vi "Step Index Assigner.vi"(0 "Parameters In":string[][](array[string]), 5 "Controller?":bool=TRUE, 7 "Flow":i32, 9 "Maxes":dbl[](array[numeric]), 11 "Mins":dbl[](array[numeric])) -> (4 "Parameters Out":string[][](array[string]), 6 "Valid?":bool, 8 "TimeValid?":bool, 10 "ProfileValid?":bool, 15 "NoCoerces":bool)   [LabVIEW 2013]
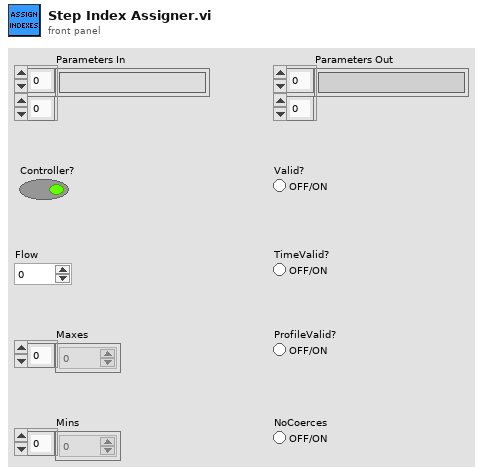
[diagram p1: front panel]
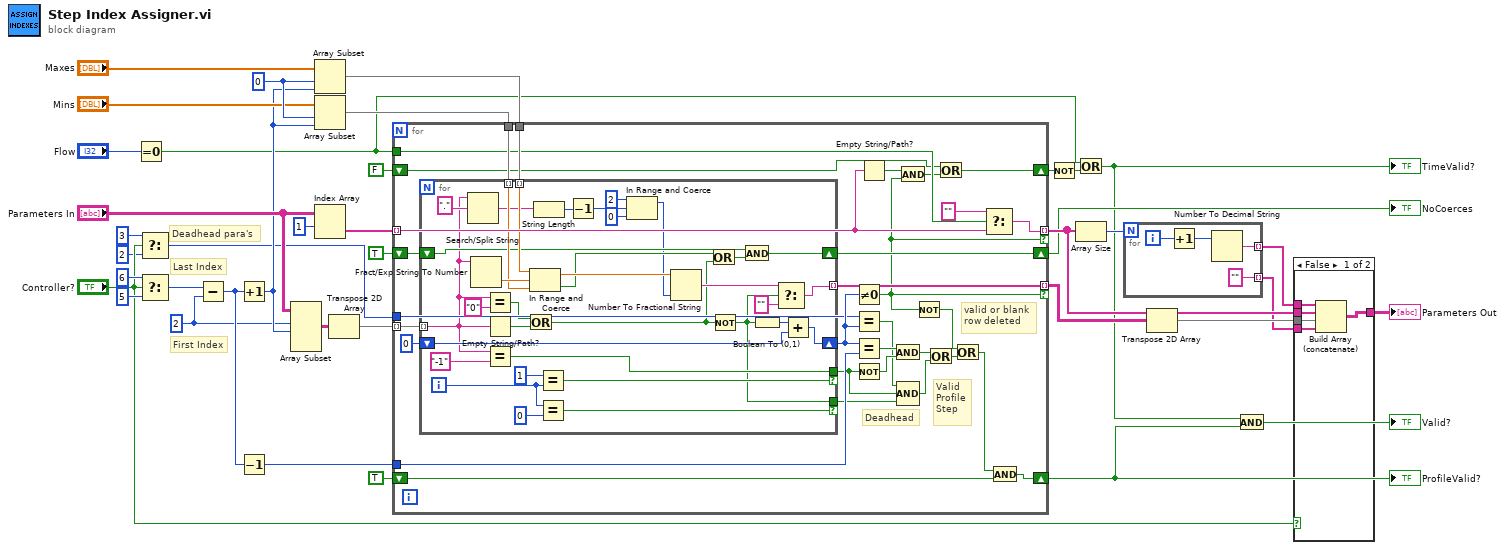
[diagram p0: block diagram]
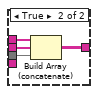
[diagram p2: hidden frame]
diagram:
  w9 = 2 ("y")
  w34 = 0 ("index")
  # "Deadhead para's"
  # "First Index"
  # "Last Index"
  n1 = Equal To 0?(x="Flow") -> (x = 0?=w10:bool)
  n2 = Select(t=3, s="Controller?", f=2) -> (s? t:f=w1:i32)
  n3 = Select(t=6, s="Controller?", f=5) -> (s? t:f=w37:i32)
  n4 = Subtract(x=w37, y=w9) -> (x-y=w36:i32)
  n5 = Increment(x=w36) -> (x+1=w16:i32)
  n6 = Decrement(x=w36) -> (x-1=w35:i32)
  n7 = Array Subset(array="Parameters In", index (row)=w9, length (row)=w16) -> (w27:string[][])  [unwired: 2 in]
  n8 = Array Subset(array="Maxes", index=w34, length=w16) -> (w31:dbl[])
  n9 = Array Subset(array="Mins", index=w34, length=w16) -> (w30:dbl[])
  n10 = Index Array(array="Parameters In", index (row)=1) -> (element=w25:string[])  [unwired: 1 in]
  n11 = Transpose 2D Array(2D array=w27) -> (transposed array=w26:string[][])
  n12 = for {
    tunnel: w26 -> [w69] mode=indexing
    tunnel: w35 -> [w68]
    tunnel: [w63] -> w21 mode=indexing if=w43
    tunnel: w31 -> [w67]
    tunnel: w30 -> [w66]
    shift-right: [w64] -> w7
    shift-left: TRUE -> [w65]
    tunnel: [w62] -> w22 mode=indexing if=w43
    tunnel: w25 -> [w55] mode=indexing
    tunnel: w10 -> [w61]
    shift-right: [w59] -> w8
    shift-left: TRUE -> [w58]
    shift-right: [w54] -> w12
    shift-left: FALSE -> [w41]
    tunnel: w1 -> [w40]
    # "valid or blank\nrow deleted"
    # "Valid\nProfile\nStep"
    # "Deadhead"
    n13 = for {
      tunnel: w69 -> [w73] mode=indexing
      shift-right: [w102] -> w49
      shift-left: i16 0 -> [w103]
      tunnel: [w100] -> w53 if=w98
      tunnel: [w88] -> w63 mode=indexing
      tunnel: w67 -> [w95] mode=indexing
      tunnel: w66 -> [w94] mode=indexing
      shift-right: [w92] -> w64
      shift-left: w65 -> [w93]
      tunnel: [w71] -> w57 if=w72
      i -> [w75]
      n14 = Search/Split String(string=w73, search string/char (-)="." ("regular expression")) -> (match + rest of string=w85:string)  [unwired: 1 in, 2 out]
      n15 = Fract/Exp String To Number(string=w73) -> (number=w97:dbl)  [unwired: 3 in, 1 out]
      n16 = Equal?(x=w73, y="0") -> (x = y?=w78:bool)
      n17 = Empty String/Path?(string/path=w73) -> (empty?=w77:bool)
      n18 = Equal?(x=w73, y="-1") -> (x = y?=w100:bool)
      n19 = Or(x=w78, y=w77) -> (x .or. y?=w76:bool)
      n20 = In Range and Coerce(upper limit=w95, x=w97, lower limit=w94) -> (coerced(x)=w96:dbl, In Range?=w91:bool)
      n21 = String Length(string=w85) -> (length=w84:i32)
      n22 = Equal?(x=1, y=w75) -> (x = y?=w98:bool)
      n23 = Equal?(x=w75, y=0 ("x")) -> (x = y?=w72:bool)
      n24 = Decrement(x=w84) -> (x-1=w83:i32)
      n25 = In Range and Coerce(upper limit=2, x=w83, lower limit=0) -> (coerced(x)=w82:i32)  [unwired: 1 out]
      n26 = Number To Fractional String(number=w96, precision (6)=w82) -> (F-format string=w89:string)  [unwired: 2 in]
      n27 = Or(x=w91, y=w76) -> (x .or. y?=w90:bool)
      n28 = Not(x=w76) -> (.not. x?=w71:bool)
      n29 = And(x=w93, y=w90) -> (x .and. y?=w92:bool)
      n30 = Boolean To (0,1)(Boolean=w71) -> (0, 1=w104:i16)
      n31 = Select(t=w89, s=w71, f="") -> (s? t:f=w88:string)
      n32 = Add(x=w104, y=w103) -> (x+y=w102:i16)
    }
    n33 = Not Equal To 0?(x=w49) -> (x != 0?=w43:bool)
    n34 = Equal?(x=w40, y=w49) -> (x = y?=w48:bool)
    n35 = Equal?(x=w49, y=w68) -> (x = y?=w51:bool)
    n36 = Not(x=w53) -> (.not. x?=w52:bool)
    n37 = Empty String/Path?(string/path=w55) -> (empty?=w44:bool)
    n38 = And(x=w51, y=w52) -> (x .and. y?=w50:bool)
    n39 = Compound Arithmetic op=AND(w48, w53, w57) -> (w56:bool)
    n40 = And(x=w44, y=w43) -> (x .and. y?=w42:bool)
    n41 = Not(x=w43) -> (.not. x?=w47:bool)
    n42 = Or(x=w50, y=w56) -> (x .or. y?=w46:bool)
    n43 = Or(x=w41, y=w42) -> (x .or. y?=w54:bool)
    n44 = Or(x=w47, y=w46) -> (x .or. y?=w45:bool)
    n45 = Select(t="", s=w61, f=w55) -> (s? t:f=w62:string)
    n46 = And(x=w45, y=w58) -> (x .and. y?=w59:bool)
  }
  "NoCoerces" <- w7
  "ProfileValid?" <- w8
  n47 = Not(x=w12) -> (.not. x?=w11:bool)
  n48 = Or(x=w10, y=w11) -> (x .or. y?=w6:bool)
  "TimeValid?" <- w6
  n49 = Array Size(array=w22) -> (size(s)=w24:i32)
  n50 = for {
    N: w24 -> [_]
    tunnel: [w106] -> w23 mode=indexing
    tunnel: ["" ("t")] -> w19 mode=indexing
    i -> [w108]
    n51 = Increment(x=w108) -> (x+1=w107:i32)
    n52 = Number To Decimal String(number=w107) -> (decimal integer string=w106:string)  [unwired: 1 in]
  }
  n53 = Transpose 2D Array(2D array=w21) -> (transposed array=w20:string[][])
  n54 = And(x=w6, y=w8) -> (x .and. y?=→"Valid?":bool)
  n55 = case shown="False" "Controller?" {
    tunnel: w23 -> [w113 w117]
    tunnel: w22 -> [w112 w116]
    tunnel: w20 -> [w111 w115]
    tunnel: w19 -> [w110 _]
    tunnel: [w109 w114] -> w18
    frame False {
      n56 = Build Array (concatenate)(w113, w112, w111, w110) -> (w109:string[][])
    }
    frame True {
      n57 = Build Array (concatenate)(w117, w116, w115) -> (w114:string[][])
    }
  }
  "Parameters Out" <- w18
